vi "Reset_FPGA_Module.vi"(8 "error in (no error)":errorcluster, 11 "connection ID":refnum<k5>) -> (0 "error out":errorcluster, 3 "connection ID out":refnum<k5>, 4 "Answer to Reset":string)   [LabVIEW 2015, in "VIPM2.lvlib"]
uses:
  VIPM2.lvlib
panel:
  # "MODULE FPGA RESET"
  # "Resets the FPGAs of all layers and all its chips."
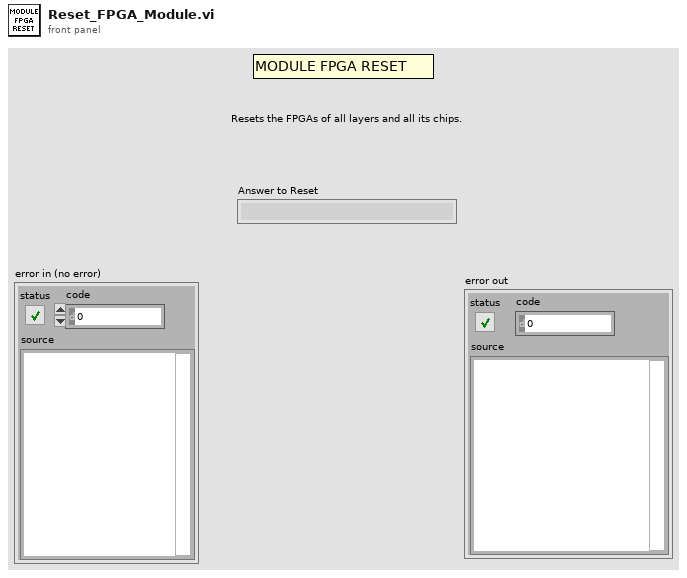
[diagram p1: front panel]
types:
  T1 = enum16{"Standard", "Buffered", "CRLF", "Immediate"}
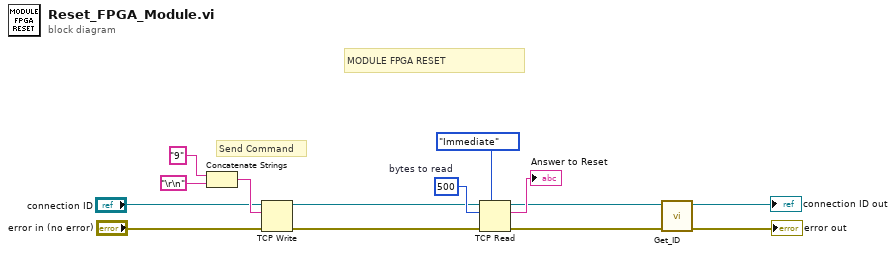
[diagram p0: block diagram]
diagram:
  w8 = 500  # bytes to read
  # "Send Command"
  # "MODULE FPGA RESET"
  n1 = Concatenate Strings("9" ("string"), "\r\n") -> (w12:string)
  n2 = TCP Write(connection ID="connection ID", data in=w12, error in (no error)="error in (no error)") -> (connection ID out=w7:refnum<k5>, error out=w6:errorcluster)  [unwired: 1 in, 1 out]
  n3 = TCP Read(connection ID=w7, bytes to read=w8, error in (no error)=w6, 7:T1."Immediate" ("mode (standard)")) -> (connection ID out=w4:refnum<k5>, data out=→"Answer to Reset":string, error out=w3:errorcluster)  [unwired: 1 in]
  n4 = call "Get_ID.vi"("error in (no error)"=w3, "connection ID"=w4) -> ("error out"=→"error out":errorcluster, "connection ID out"=→"connection ID out":refnum<k5>)  [unwired: 6 in, 2 out]
